vi "Write Data Source Type.vi"(8 "error in (no error)":errorcluster, 10 "Data Source Type":string, 11 "DatabaseBaseClass in":refnum<class "DatabaseBaseClass.lvclass">) -> (0 "error out":errorcluster, 3 "DatabaseBaseClass out":refnum<class "DatabaseBaseClass.lvclass">)   [LabVIEW 2018, in "Database.lvlib" / "DatabaseBaseClass.lvclass"]
uses:
  DatabaseBaseClass.lvclass
  DatabaseBaseClass.lvclass/DatabaseBaseClass.ctl
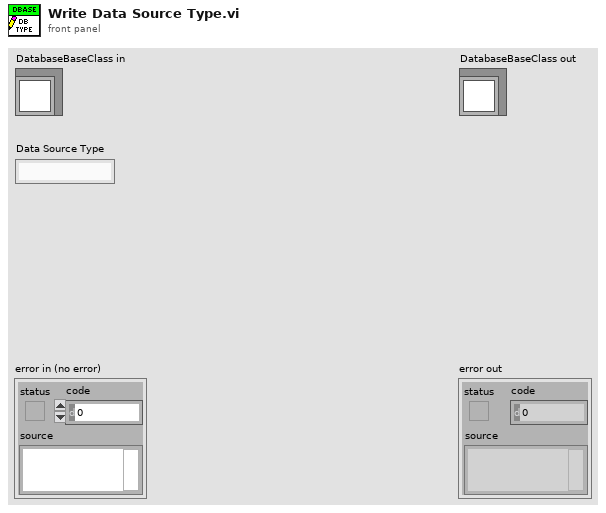
[diagram p1: front panel]
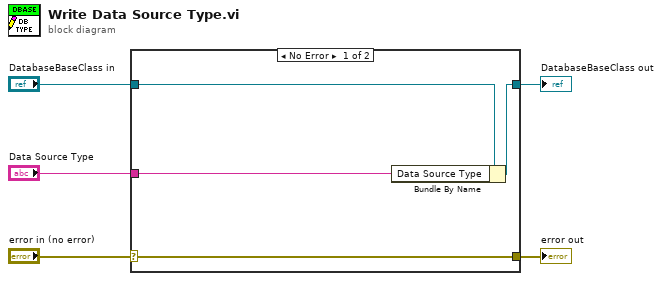
[diagram p0: block diagram]
diagram:
  n1 = case shown="No Error" "error in (no error)" {
    selector: "error in (no error)" -> [w9 w10]
    tunnel: [w9 w10] -> w4
    tunnel: [w7 w11] -> w2
    tunnel: "DatabaseBaseClass in" -> [w8 w11]
    tunnel: "Data Source Type" -> [w6 _]
    frame No Error {
      n2 = Bundle By Name(cluster=w8, "Data Source Type"=w6) -> (w7:refnum<class "DatabaseBaseClass.lvclass">)
    }
    frame Error {
    }
  }
  "error out" <- w4
  "DatabaseBaseClass out" <- w2
